vi "Inverse Real FFT(half complex).vi"(0 "FFT {X}":dbl[](array[numeric]) format="%0.2f") -> (1 "X":dbl[](array[numeric]) format="%0.2f", 2 "error":i32)   [LabVIEW 2010, in "NI_AALPro.lvlib"]
doc: "Computes the Real Fast Fourier Transform (FFT) or the Real Discrete Fourier Transform (DFT) of the input sequence <B>X</B>."
uses:
  NI_AALPro.lvlib
  lvanlys.dll
panel:
  # "Inverse Real FFT (Half Complex)"
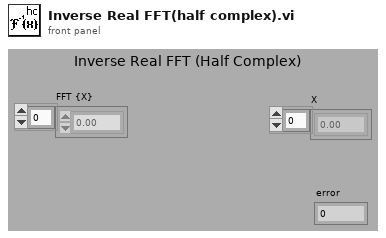
[diagram p1: front panel]
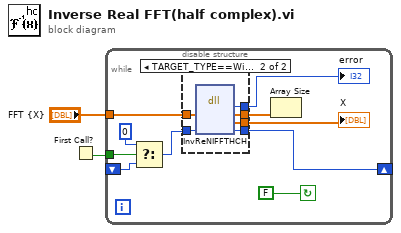
[diagram p0: block diagram]
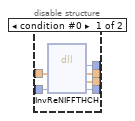
[diagram p2: hidden frame]
diagram:
  n1 = First Call?() -> (First Call?: T/F=w1:bool)
  n2 = while {
    shift-left: _ -> [w3]
    shift-right: [w5] -> _
    tunnel: "FFT {X}" -> [w12]
    tunnel: w1 -> [w4]
    stop <- FALSE continue-if-true
    n3 = Select(t=0, s=w4, f=w3) -> (s? t:f=w6:i64)
    n4 = disable-structure shown="TARGET_TYPE==Windows||TARGET_TYPE==Mac||TARGET_TYPE==Unix" {
      disable-tunnel: w12 -> [w18 w24]
      disable-tunnel: [w17 w23] -> w11
      disable-tunnel: [w16 w22] -> w10
      disable-tunnel: [w15 w21] -> w8
      disable-tunnel: w6 -> [w14 w20]
      disable-tunnel: [w13 w19] -> w5
      frame condition #0 {
        n5 = dll-call lib="C:/Program Files/National Instruments/LabVIEW 2010/resource/lvanlys.dll" fn="InvReNIFFTHCH"("xH"=w18, "arg3"=w14) -> ("return type"=w17:i32, "xH"=w15:dbl[], "yH"=w16:dbl[], "arg3"=w13:i32)  [unwired: 4 in, 2 out]
      }
      frame condition #1 (active) {
        n6 = dll-call lib="C:/Program Files/National Instruments/LabVIEW 2010/resource/lvanlys.dll" fn="InvReNIFFTHCH"("xH"=w24, "arg3"=w20) -> ("return type"=w23:i32, "xH"=w21:dbl[], "yH"=w22:dbl[], "arg3"=w19:i64)  [unwired: 4 in, 2 out]
      }
    }
    "X" <- w10
    "error" <- w11
    n7 = Array Size(array=w8) -> ()  [unwired: 1 out]
  }
